vi "Get Object by Type.vi"(7 "Object Type":refnum<class>, 8 "error in (no error)":errorcluster, 11 "Values in":refnum<class "Values.lvclass">) -> (0 "error out":errorcluster, 2 "Object":refnum<class>, 3 "Values out":refnum<class "Values.lvclass">)   [LabVIEW 2020, in "HTTP Server.lvlib" / "Values.lvclass"]
uses:
  Values.lvclass
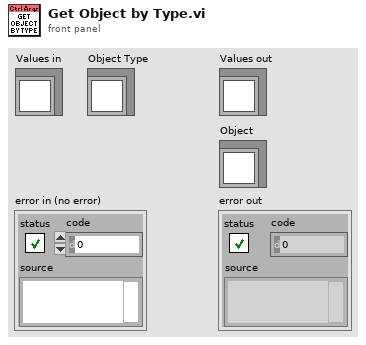
[diagram p1: front panel]
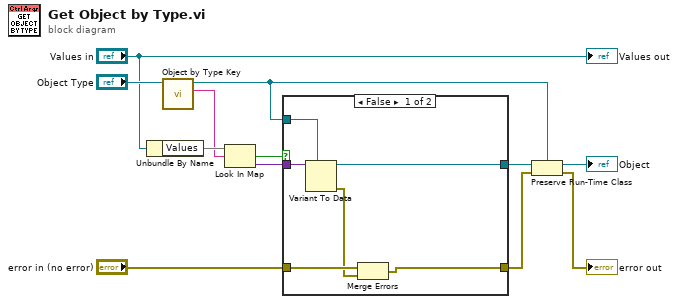
[diagram p0: block diagram]
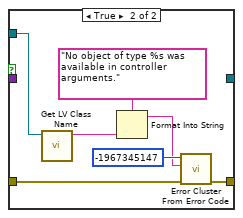
[diagram p2: hidden frame]
diagram:
  n1 = Unbundle By Name("Values in") -> ("Values"=w12:map{string, variant})
  n2 = call "Object by Type Key.vi"("Object In"="Object Type") -> ("Object Type Key"=w11:string, "Object"=w7:refnum<class>)  [unwired: 9 in]
  n3 = Look In Map(map=w12, key=w11) -> (key not found?=w10:bool, value=w9:variant)  [unwired: 1 in]
  n4 = case shown="False" w10 {
    tunnel: w9 -> [w18 _]
    tunnel: "error in (no error)" -> [w15 w22]
    tunnel: [w13 w21] -> w6
    tunnel: w7 -> [w17 w19]
    tunnel: [w16 _] -> w8
    frame False {
      n5 = Variant To Data(type=w17, Variant=w18) -> (data=w16:refnum<class>, error out=w14:errorcluster)  [unwired: 1 in]
      n6 = Merge Errors(w15, w14) -> (w13:errorcluster)
    }
    frame True {
      n7 = call <vilib>:"Get LV Class Name.vi"("object"=w19) -> ("class name"=w20:string)  [unwired: 9 in, 1 out]
      n8 = Format Into String(format string="No object of type %s was available in controller arguments.", w20) -> (resulting string=w24:string)  [unwired: 2 in, 1 out]
      n9 = call <vilib>:"Error Cluster From Error Code.vi"("error in (no error)"=w22, "error message (\"\")"=w24, "error code (0)"=-1967345147) -> ("error out"=w21:errorcluster)  [unwired: 6 in]
    }
  }
  n10 = Preserve Run-Time Class(object in=w8, error in=w6, 2:w7) -> (object out=→"Object":refnum<class>, error out=→"error out":errorcluster)
  "Values out" <- "Values in"
